vi "GET_Speed-based_density_map.vi"(0 "ImageSize":cluster{"x":i32, "y":i32}, 1 "Input array is image? (F)":bool, 5 "XY data":cluster{"Numeric":dbl, "Numeric":dbl}[](array[cluster]), 7 "Log2-transform? (T)":bool=TRUE, 9 "Normalize to 8 bit? (T)":bool=TRUE, 11 "error in (no error)":errorcluster, 12 "Output as Image? (F)":bool, 13 "Loaded.speed":dbl[](array[numeric])) -> (4 "Array or 8-bit pixmap out":u32[][](array[numeric]), 15 "error out":errorcluster)   [LabVIEW 2018, in "Tracker.lvlib"]
uses:
  Tracker.lvlib
  Controls/CTL_2D_bins_parameters.ctl
  Controls/CTL_Color_ramp.ctl
  GET_2D_Data_Binning_(additional_data).vi
panel:
  out "Interp. size":i32[](array[numeric])
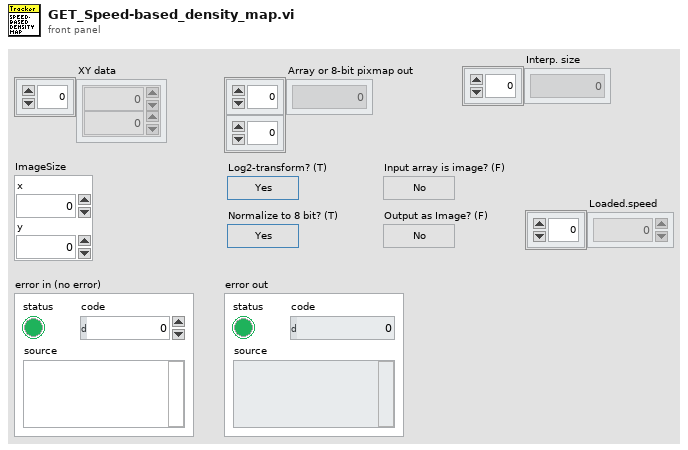
[diagram p1: front panel]
types:
  T1 = typedef "Tracker.lvlib/CTL_2D_bins_parameters.ctl" = cluster{"Xmax":dbl, "Xmin":dbl, "Ymax":dbl, "Ymin":dbl, "# bins per axis":i32}
  T2 = typedef "Tracker.lvlib/CTL_Color_ramp.ctl" = u32[]
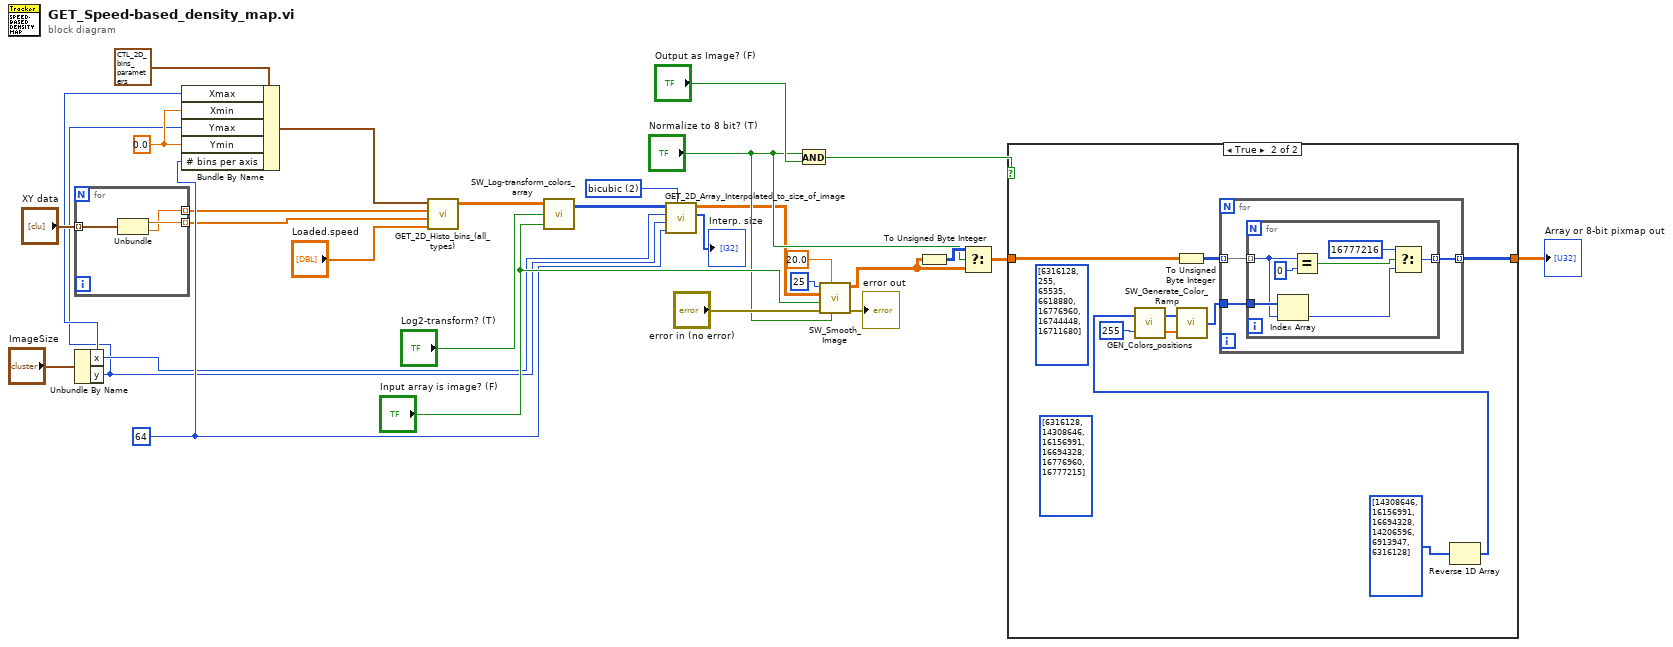
[diagram p0: block diagram]
diagram:
  w18 = 2 items=["nearest", "bilinear", "bicubic", "bicubic spline"] ("Method")
  w17 = 64 ("# bins per axis")
  w22 = 0.0 ("Xmin")
  n1 = for {
    tunnel: "XY data" -> [w32] mode=indexing
    tunnel: [w31] -> w3 mode=indexing
    tunnel: [w30] -> w2 mode=indexing
    n2 = Unbundle(w32) -> ("Numeric"=w31:dbl, "Numeric"=w30:dbl)
  }
  n3 = Unbundle By Name("ImageSize") -> ("x"=w5:i32, "y"=w4:i32)
  n4 = Bundle By Name(cluster=T1 {"Xmax"=110.0, "Xmin"=-110.0, "Ymax"=110.0, "Ymin"=-110.0, "# bins per axis"=64} ("Bins parameters"), "Xmax"=w5, "Xmin"=w22, "Ymax"=w4, "Ymin"=w22, "# bins per axis"=w17) -> (w23:T1)
  n5 = call-poly "GET_2D_Histo_bins_(all_types).vi"("Additional data"="Loaded.speed", "Y"=w3, "X"=w2, "Bins parameters"=w23) -> ("Binned array"=w9:dbl[][])  [unwired: 2 in]
  n6 = call "SW_Log-transform_colors_array.vi"("Image? (T)"="Input array is image? (F)", "Log-transform? (F)"="Log2-transform? (T)", "Array or 24-bit pixmap in"=w9) -> ("Array or 24-bit pixmap out"=w8:u32[][])  [unwired: 1 in]
  n7 = call "GET_2D_Array_Interpolated_to_size_of_image.vi"("Method"=w18, "# bins per axis"=w17, "Y image size"=w4, "X image size"=w5, "Array or pixmap in"=w8) -> ("Interp. size"=→"Interp. size":i32[], "Array or pixmap out"=w7:dbl[][])  [unwired: 5 in]
  n8 = And(x="Normalize to 8 bit? (T)", y="Output as Image? (F)") -> (x .and. y?=w11:bool)
  n9 = call "SW_Smooth_Image.vi"("Normalize to 8-bit range? (T)"="Normalize to 8 bit? (T)", "Sigma"=20.0, "Error In"="error in (no error)", "Image? (T)"="Input array is image? (F)", "Array or pixmap in"=w7, "Kernel size"=u32 25) -> ("Error Out"=→"error out":errorcluster, "Array or pixmap out"=w6:dbl[][])  [unwired: 4 in]
  n10 = To Unsigned Byte Integer(number=w6) -> (unsigned 8bit integer=w15:u8[][])
  n11 = Select(t=w15, s="Normalize to 8 bit? (T)", f=w6) -> (s? t:f=w12:dbl[][])
  n12 = case shown="True" w11 {
    tunnel: [w33 w36] -> w13
    tunnel: w12 -> [w33 w42]
    frame False {
    }
    frame True {
      (unwired) u32[] [6316128, 14308646, 16156991, 16694328, 16776960, 16777215] ("Initial colors ramp array")
      (unwired) T2 [6316128, 255, 65535, 6618880, 16776960, 16744448, 16711680] ("Initial colors ramp array")
      n13 = To Unsigned Byte Integer(number=w42) -> (unsigned 8bit integer=w39:u8[][])
      n14 = Reverse 1D Array(array=u32[] [14308646, 16156991, 16694328, 14206596, 6913947, 6316128] ("Initial colors ramp array")) -> (reversed array=w34:u32[])
      n15 = call "GEN_Colors_positions.vi"("Highest color position"=u32 255, "Initial colors ramp array in"=w34) -> ("Colors positions"=w41:dbl[], "Initial colors ramp array out"=w40:T2)
      n16 = call "SW_Generate_Color_Ramp.vi"("Colors rel. pos."=w41, "Colors array"=w40) -> ("Colors array"=w37:u32[])
      n17 = for {
        tunnel: w39 -> [w45] mode=indexing
        tunnel: [w44] -> w36 mode=indexing
        tunnel: w37 -> [w43]
        n18 = for {
          tunnel: w45 -> [w49] mode=indexing
          tunnel: [w46] -> w44 mode=indexing
          tunnel: w43 -> [w52]
          n19 = Index Array(array=w52, index=w49) -> (element=w47:u32)
          n20 = Equal?(x=w49, y=0) -> (x = y?=w50:bool)
          n21 = Select(t=16777216, s=w50, f=w47) -> (s? t:f=w46:u32)
        }
      }
    }
  }
  "Array or 8-bit pixmap out" <- w13
